vi "get_channel_colours.vi"(8 "error in (no error)":errorcluster, 11 "DL090216Display.lvclass in":refnum<class "DisplayDL090216.lvclass">) -> (0 "error out":errorcluster, 2 "channel colours":T1[](array[typedef]), 3 "DL090216Display.lvclass out":refnum<class "DisplayDL090216.lvclass">)   [LabVIEW 2010, in "DisplayDL090216.lvclass"]
uses:
  DisplayDL090216.lvclass
  common/classes/Image/Image/colour_enum.ctl
  common/classes/Image/Image/Image.lvclass
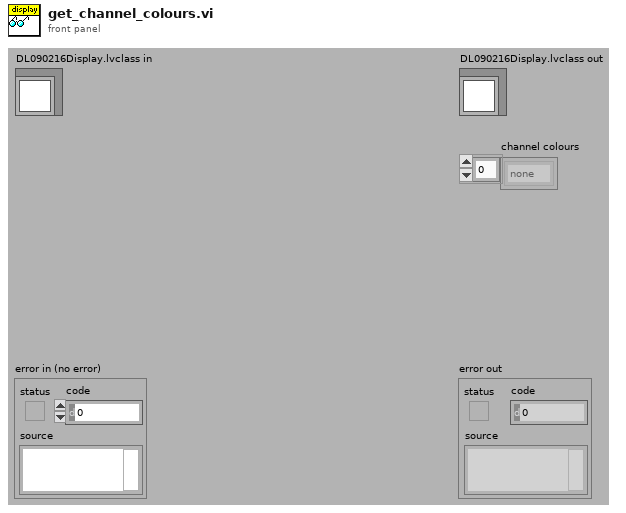
[diagram p1: front panel]
types:
  T1 = typedef "Image.lvclass/colour_enum.ctl" = enum16{"none", "red", "green", "blue", "grey scale", "custom"}
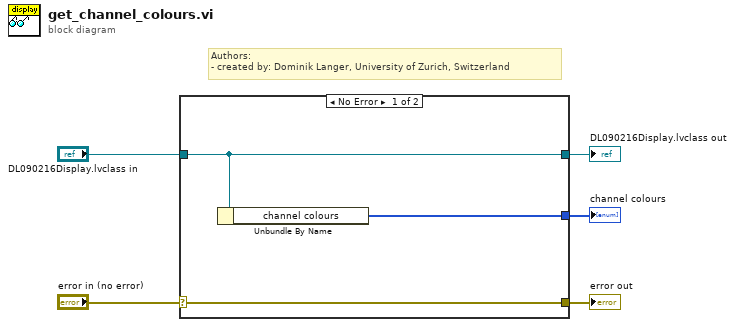
[diagram p0: block diagram]
diagram:
  # "Authors: \n- created by: Dominik Langer, University of Zurich, Switzerland"
  n1 = case shown="No Error" "error in (no error)" {
    selector: "error in (no error)" -> [w8 w9]
    tunnel: [w8 w9] -> w4
    tunnel: [w7 w10] -> w2
    tunnel: "DL090216Display.lvclass in" -> [w7 w10]
    tunnel: [w6 _] -> w1
    frame No Error {
      n2 = Unbundle By Name(w7) -> ("channel colours"=w6:T1[])
    }
    frame Error {
    }
  }
  "error out" <- w4
  "DL090216Display.lvclass out" <- w2
  "channel colours" <- w1
